vi "PID控制.vi"() -> ()   [LabVIEW 2022 SP3]
panel:
  in  "比例":dbl=5.0
  in  "微分":dbl
  in  "积分":dbl=1.0
  in  "目标值":dbl=5.0
  out "过程输出值":dbl format="%_12g"
  out "Waveform Chart":dbl(graph)
  in  "循环时间":dbl=1023.0 format="%#_3g"
  in  "初始值":dbl
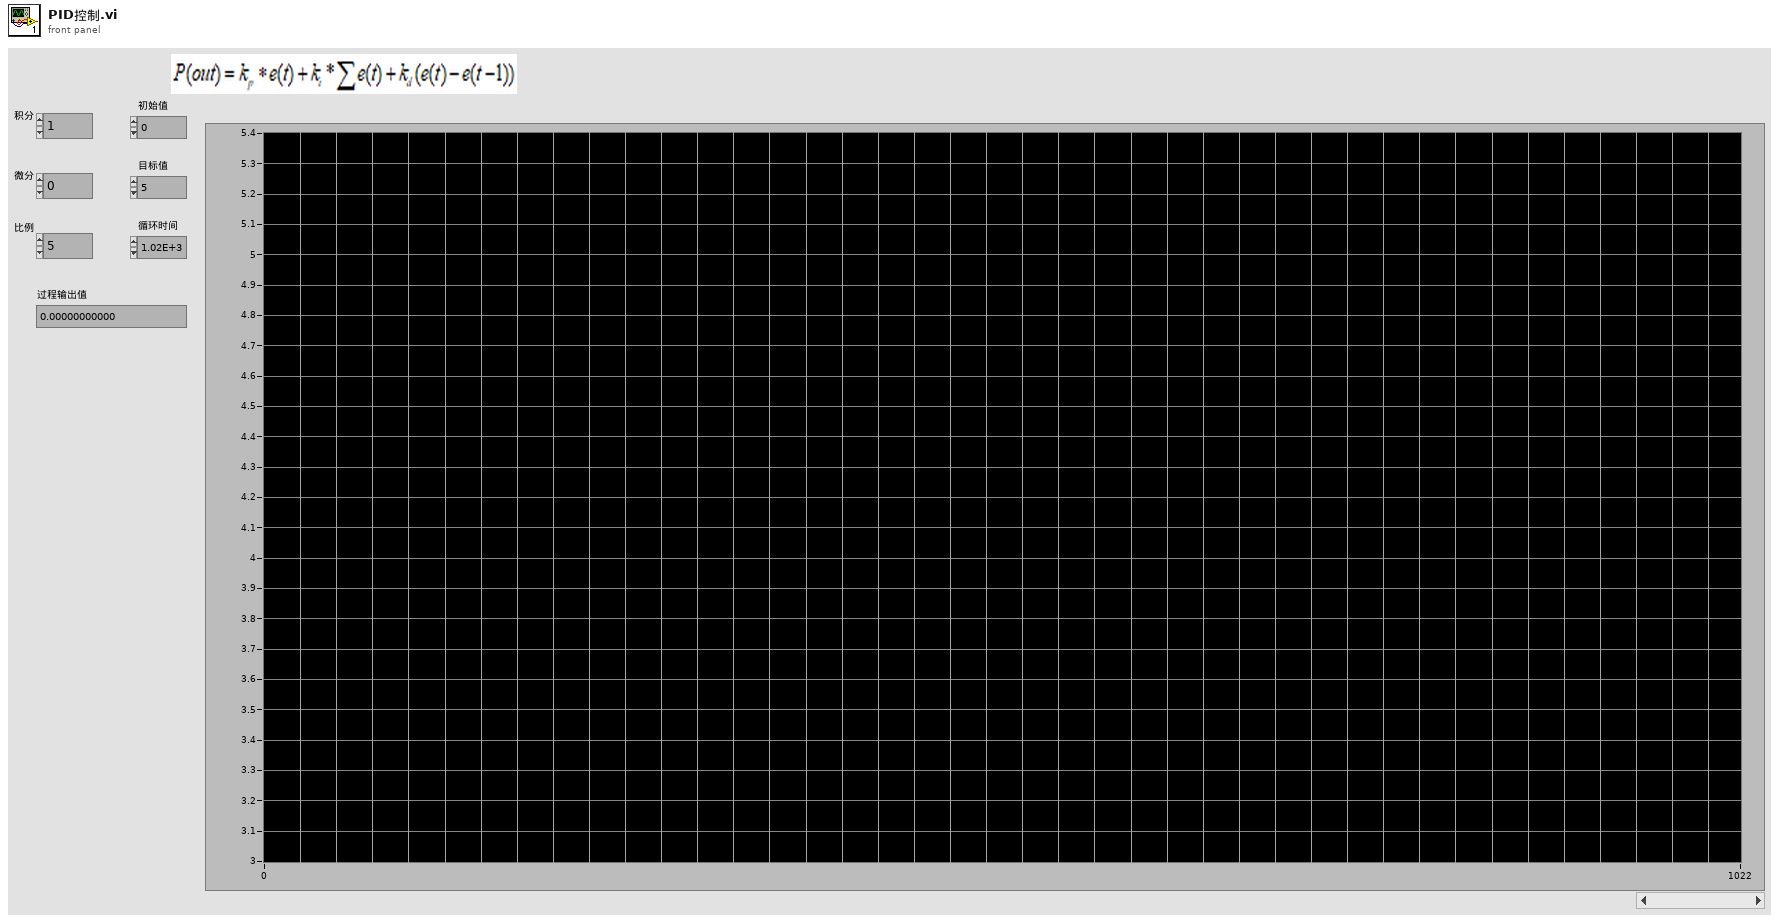
[diagram p1: front panel]
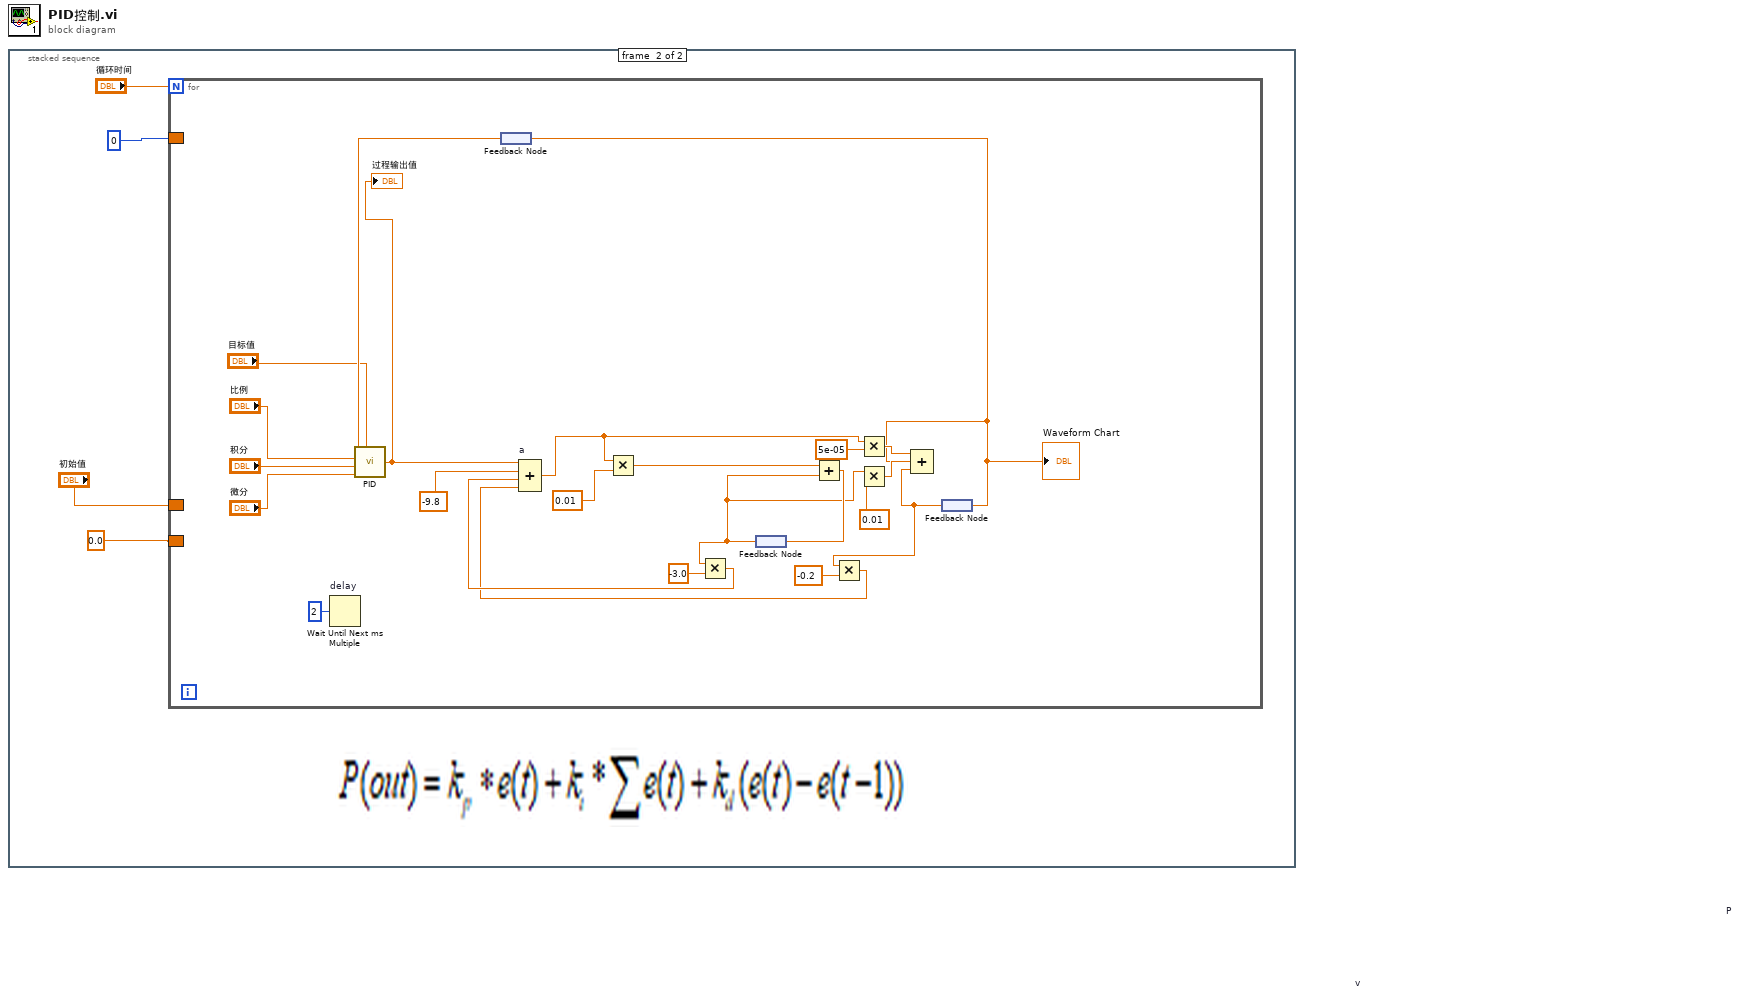
[diagram p0: block diagram]
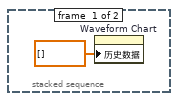
[diagram p2: hidden frame]
diagram:
  n1 = stacked-sequence {
    frame #0 {
      n2 = property on="Waveform Chart" class="WFChart (严格)"("历史数据"=dbl[] []) -> ()  [unwired: 2 in, 2 out]
    }
    frame #1 {
      n3 = for {
        N: "循环时间" -> [_]
        border: 0.0 -> [_]
        border: "初始值" -> [_]
        border: 0 -> [_]
        n4 = Wait Until Next ms Multiple "delay"(millisecond multiple=u32 2) -> ()  [unwired: 1 out]
        n5 = feedback #1() -> (w14:dbl)
        n6 = call "PID.vi"("当前值"=w14, "kp"="比例", "ki"="积分", "kd"="微分", "目标值"="目标值") -> ("输出值"=w15:dbl)
        "过程输出值" <- w15
        n7 = feedback #2 "v"() -> (w8:dbl)
        n8 = Multiply(x=w8, y=-3.0) -> (x*y=w18:dbl)
        n9 = Multiply(x=w8, y=0.01) -> (x*y=w21:dbl)
        n10 = feedback #3 "P"() -> (w10:dbl)
        n11 = Multiply(x=w10, y=-0.2) -> (x*y=w16:dbl)
        n12 = Compound Arithmetic op=ADD "a"(w15, -9.8 ("值"), w18, w16) -> (w9:dbl)
        n13 = Multiply(x=w9, y=0.01) -> (x*y=w25:dbl)
        n14 = Add(x=w25, y=w8) -> (x+y=w23:dbl)
        n15 = feedback-in #2(w23) -> ()
        n16 = Multiply(x=w9, y=5e-05) -> (x*y=w20:dbl)
        n17 = Compound Arithmetic op=ADD(w20, w21, w10) -> (w7:dbl)
        "Waveform Chart" <- w7
        n18 = feedback-in #1(w7) -> ()
        n19 = feedback-in #3(w7) -> ()
      }
    }
  }
